vi "button_pressed.vi"(1 "Button In":bool) -> (0 "Button Pressed?":bool)   [LabVIEW 2014]
panel:
  # "Boolean signal rising edge"
  # "Made this as a space-saving VI\n\nalso, it's reentrant"
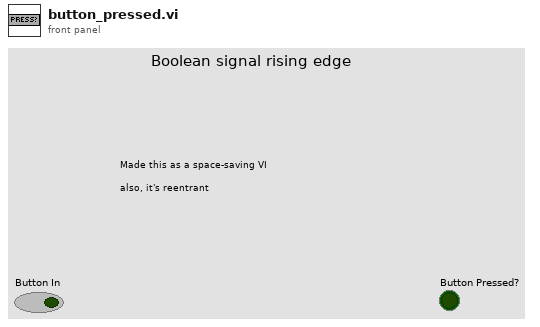
[diagram p1: front panel]
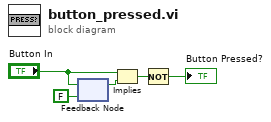
[diagram p0: block diagram]
diagram:
  n1 = feedback #1(FALSE ("Button 2")) -> (w5:bool)
  n2 = feedback-in #1("Button In") -> ()
  n3 = Implies(1:w5, 2:"Button In") -> (0:w4:bool)
  n4 = Not(x=w4) -> (.not. x?=→"Button Pressed?":bool)
